vi "FRCts20_WebMethods_ESP_Team.vi"(8 "error in (no error)":errorcluster, 9 "Team":T2, 10 "Return Type":T4="mobile", 11 "httpRequestID":u32) -> (0 "error out":errorcluster, 3 "httpRequestID out":u32)   [LabVIEW 2014, in "FRCts20_WebMethods.lvlib"]
uses:
  FRCts20_WebMethods.lvlib
  <vilib>/wsapi/NI_WebServices.lvlib
  <vilib>/wsapi/subVIs/Set Integer ESP Variable.vi
  <vilib>/wsapi/subVIs/Set String ESP Variable.vi
  Controls/FRCts20_WebMethods_Globals.vi
  Controls/FRCts20_WebMethods_ctl_returntype.ctl
  Backend/source/VI Source/FRCts20_Backend_API/FRCts20_Backend_API_SW.ctl
  Backend/source/VI Source/FRCts20_Backend_API/FRCts20_Backend_API_Status.ctl
  Backend/source/VI Source/FRCts20_Backend_API/FRCts20_Backend_API_Team.ctl
panel:
  in  "SWType (hidden)":T1
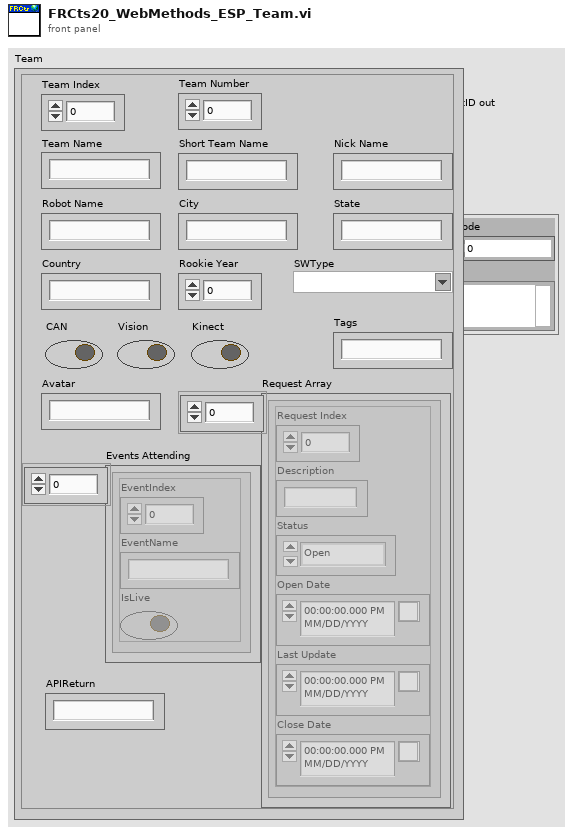
[diagram p1: front panel]
types:
  T1 = typedef "FRCts20_Backend_API.lvlib/FRCts20_Backend_API_SW.ctl" = string
  T2 = typedef "FRCts20_Backend_API.lvlib/FRCts20_Backend_API_Team.ctl" = cluster{"Team Index":u32, "Team Number":u32, "Team Name":string, "Short Team Name":string, "Nick Name":string, "Robot Name":string, "City":string, "State":string, "Country":string, "Rookie Year":u32, "SWType":T1, "CAN":bool, "Vision":bool, "Kinect":bool, "Tags":string, "Avatar":string, "Request Array":cluster{"Request Index":u32, "Description":string, "Status":T3, "Open Date":timestamp, "Last Update":timestamp, "Close Date":timestamp}[], "Events Attending":cluster{"EventIndex":dbl, "EventName":string, "IsLive":bool}[], "APIReturn":string}
  T3 = typedef "FRCts20_Backend_API.lvlib/FRCts20_Backend_API_Status.ctl" = enum16{"Open", "In Work", "Closed"}
  T4 = typedef "FRCts20_WebMethods.lvlib/FRCts20_WebMethods_ctl_returntype.ctl" = string
  T5 = cluster{"Request Index":u32, "Description":string, "Status":T3, "Open Date":timestamp, "Last Update":timestamp, "Close Date":timestamp}[]
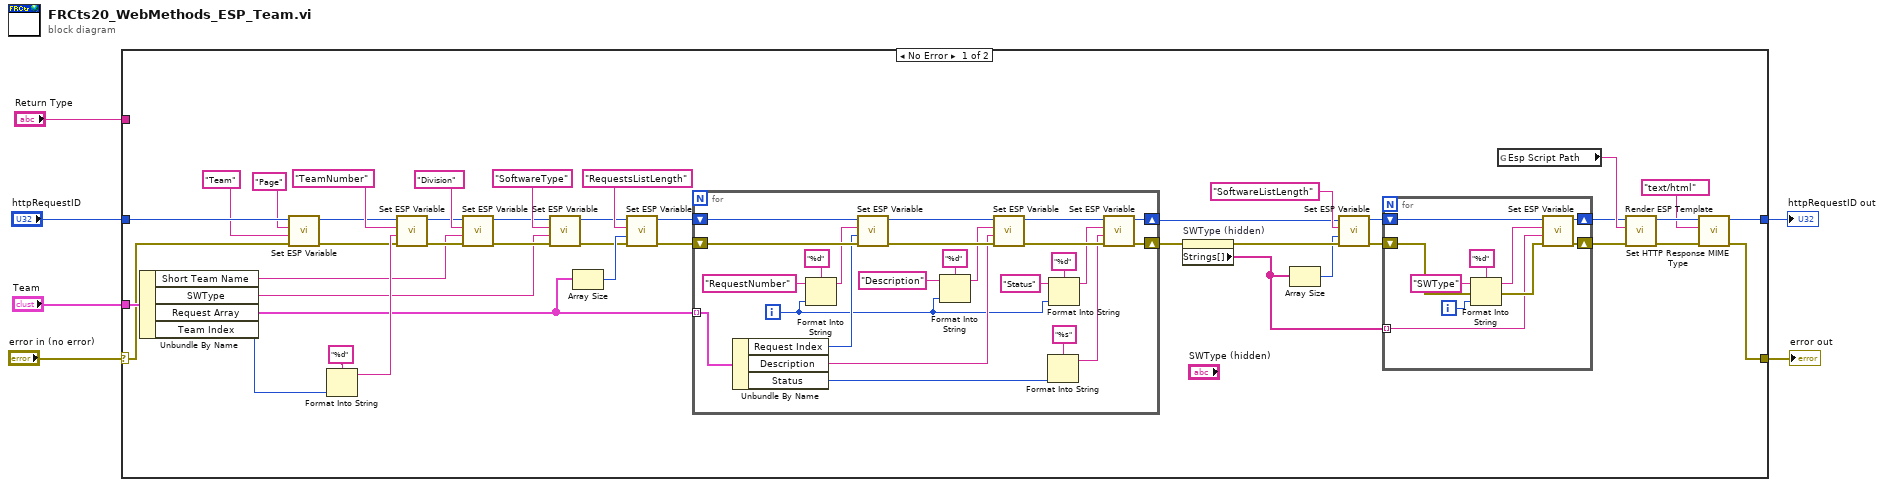
[diagram p0: block diagram]
diagram:
  n1 = case shown="No Error" "error in (no error)" {
    selector: "error in (no error)" -> [w26 w84]
    tunnel: "httpRequestID" -> [w25 w83]
    tunnel: [w46 w83] -> w3
    tunnel: [w45 w84] -> w2
    tunnel: "Return Type" -> [_ _]
    tunnel: "Team" -> [w36 _]
    frame No Error {
      n2 = Unbundle By Name(w36) -> ("Short Team Name"=w19:string, "SWType"=w18:T1, "Request Array"=w17:T5, "Team Index"=w20:u32)
      n3 = call-poly <vilib>:"Set ESP Variable.vi"("error in (no error)"=w26, "value"="Team", "key"="Page", "httpRequestID"=w25) -> ("error out"=w28:errorcluster, "httpRequestID out"=w27:u32)  [unwired: 6 in]
      n4 = Format Into String(format string="%d", w20) -> (resulting string=w31:string)  [unwired: 2 in, 1 out]
      n5 = call-poly <vilib>:"Set ESP Variable.vi"("error in (no error)"=w28, "value"=w31, "key"="TeamNumber", "httpRequestID"=w27) -> ("error out"=w32:errorcluster, "httpRequestID out"=w33:u32)  [unwired: 6 in]
      n6 = call-poly <vilib>:"Set ESP Variable.vi"("error in (no error)"=w32, "value"=w19, "key"="Division", "httpRequestID"=w33) -> ("error out"=w42:errorcluster, "httpRequestID out"=w41:u32)  [unwired: 6 in]
      n7 = call-poly <vilib>:"Set ESP Variable.vi"("error in (no error)"=w42, "value"=w18, "key"="SoftwareType", "httpRequestID"=w41) -> ("error out"=w22:errorcluster, "httpRequestID out"=w21:u32)  [unwired: 6 in]
      n8 = Array Size(array=w17) -> (size(s)=w39:i32)
      n9 = call-poly <vilib>:"Set ESP Variable.vi"("error in (no error)"=w22, "value"=w39, "key"="RequestsListLength", "httpRequestID"=w21) -> ("error out"=w40:errorcluster, "httpRequestID out"=w37:u32)  [unwired: 6 in]
      n10 = for {
        shift-right: [w69] -> w10
        shift-left: w40 -> [w82]
        tunnel: w17 -> [w77] mode=indexing
        shift-right: [w68] -> w9
        shift-left: w37 -> [w78]
        i -> [w63]
        n11 = Unbundle By Name(w77) -> ("Request Index"=w76:u32, "Description"=w71:string, "Status"=w60:T3)
        n12 = Format Into String(format string="%d", initial string="RequestNumber", w63) -> (resulting string=w80:string)  [unwired: 1 in, 1 out]
        n13 = call-poly <vilib>:"Set ESP Variable.vi"("error in (no error)"=w82, "value"=w76, "key"=w80, "httpRequestID"=w78) -> ("error out"=w75:errorcluster, "httpRequestID out"=w74:u32)  [unwired: 6 in]
        n14 = Format Into String(format string="%d", initial string="Description", w63) -> (resulting string=w70:string)  [unwired: 1 in, 1 out]
        n15 = call-poly <vilib>:"Set ESP Variable.vi"("error in (no error)"=w75, "value"=w71, "key"=w70, "httpRequestID"=w74) -> ("error out"=w66:errorcluster, "httpRequestID out"=w67:u32)  [unwired: 6 in]
        n16 = Format Into String(format string="%s", w60) -> (resulting string=w59:string)  [unwired: 2 in, 1 out]
        n17 = Format Into String(format string="%d", initial string="Status", w63) -> (resulting string=w62:string)  [unwired: 1 in, 1 out]
        n18 = call-poly <vilib>:"Set ESP Variable.vi"("error in (no error)"=w66, "value"=w59, "key"=w62, "httpRequestID"=w67) -> ("error out"=w69:errorcluster, "httpRequestID out"=w68:u32)  [unwired: 6 in]
      }
      n19 = property on="SWType (hidden)" class="CmbBox (strict)"(error in=w10) -> (error out=w16:errorcluster, "Strings[]"=w15:string[])  [unwired: 1 in, 1 out]
      n20 = Array Size(array=w15) -> (size(s)=w14:i32)
      n21 = call-poly <vilib>:"Set ESP Variable.vi"("error in (no error)"=w16, "value"=w14, "key"="SoftwareListLength", "httpRequestID"=w9) -> ("error out"=w12:errorcluster, "httpRequestID out"=w11:u32)  [unwired: 6 in]
      n22 = for {
        shift-right: [w58] -> w7
        shift-left: w12 -> [w51]
        shift-right: [w52] -> w8
        shift-left: w11 -> [w57]
        tunnel: w15 -> [w49] mode=indexing
        i -> [w55]
        n23 = Format Into String(format string="%d", initial string="SWType", error in=w51, w55) -> (resulting string=w54:string, error out=w50:errorcluster)
        n24 = call-poly <vilib>:"Set ESP Variable.vi"("error in (no error)"=w50, "value"=w49, "key"=w54, "httpRequestID"=w57) -> ("error out"=w58:errorcluster, "httpRequestID out"=w52:u32)  [unwired: 6 in]
      }
      n25 = global read "FRCts20_WebMethods_Globals.vi" "Esp Script Path"() -> (w35:string)
      n26 = call <vilib>:"Render ESP Template.vi"("error in (no error)"=w7, "espName"=w35, "httpRequestID"=w8) -> ("error out"=w47:errorcluster, "httpRequestID out"=w48:u32)  [unwired: 7 in]
      n27 = call <vilib>:"Set HTTP Response MIME Type.vi"("error in (no error)"=w47, "MIME type (text/html)"="text/html", "httpRequestID"=w48) -> ("error out"=w45:errorcluster, "httpRequestID out"=w46:u32)  [unwired: 7 in]
    }
    frame Error {
    }
  }
  "httpRequestID out" <- w3
  "error out" <- w2
